vi "Create.vi"(8 "error in (no error)":errorcluster, 10 "gRPC ID in":T1) -> (0 "error out":errorcluster, 2 "gRPC ID out":T1, 3 "IMeasurementService out":refnum<class "IMeasurementService.lvclass">)   [LabVIEW 2020, in "MeasurementLink Measurement Server.lvlib" / "MeasurementServiceV2.lvclass"]
uses:
  MeasurementServiceV2.lvclass
  IMeasurementService/IMeasurementService.lvclass
  <vilib>/gRPC/LabVIEW gRPC Library/Shared/grpcId.ctl
  MeasurementLink Measurement Service Base V2/RPC Service/MeasurementService/MeasurementServiceBaseV2.lvclass
  \\tsclient\C/dev/measurementlink-labview/Source/Runtime/MeasurementLink Measurement Server/Classes/IMeasurementService/IMeasurementService.lvclass
  MeasurementServiceV2.lvclass/MeasurementServiceV2.ctl
  <vilib>/gRPC/LabVIEW gRPC Library/grpc-lvsupport-release.lvlib
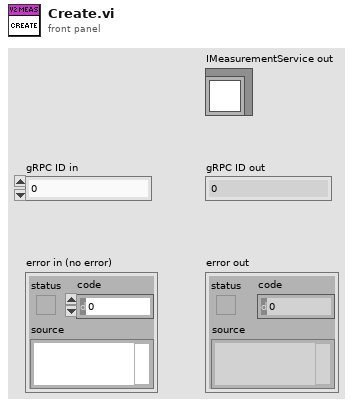
[diagram p1: front panel]
types:
  T1 = typedef "grpc-lvsupport-release.lvlib/grpcId.ctl" = u64
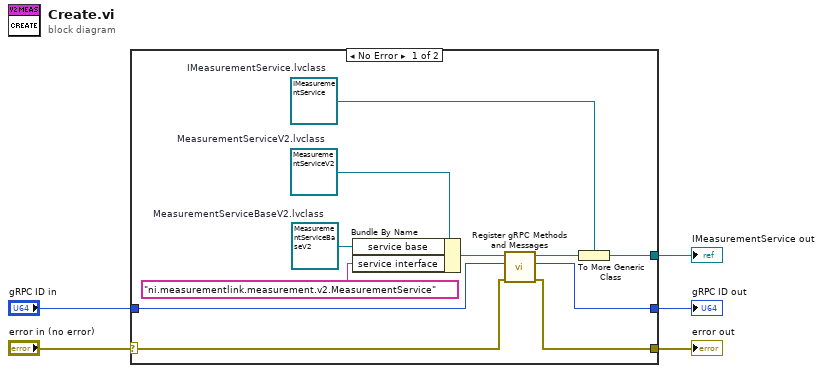
[diagram p0: block diagram]
diagram:
  n1 = case shown="No Error" "error in (no error)" {
    selector: "error in (no error)" -> [w8 w18]
    tunnel: [w7 w18] -> w4
    tunnel: [w14 _] -> w3
    tunnel: "gRPC ID in" -> [w9 w17]
    tunnel: [w6 w17] -> w1
    frame No Error {
      w12 = refnum<class "MeasurementServiceV2.lvclass"> refnum  # MeasurementServiceV2.lvclass
      w13 = refnum<class "IMeasurementService.lvclass"> refnum  # IMeasurementService.lvclass
      w16 = refnum<class "MeasurementServiceBaseV2.lvclass"> refnum  # MeasurementServiceBaseV2.lvclass
      n2 = Bundle By Name(cluster=w12, "service base"=w16, "service interface"="ni.measurementlink.measurement.v2.MeasurementService") -> (w11:refnum<class "MeasurementServiceV2.lvclass">)
      n3 = call "Register gRPC Methods and Messages.vi"("error in (no error)"=w8, "gRPC ID in"=w9, "MeasurementServiceV2 in"=w11) -> ("error out"=w7:errorcluster, "gRPC ID out"=w6:T1, "MeasurementServiceV2 out"=w10:refnum<class "MeasurementServiceV2.lvclass">)  [unwired: 6 in]
      n4 = To More Generic Class(target class=w13, reference=w10) -> (generic class reference=w14:refnum<class "IMeasurementService.lvclass">)
    }
    frame Error {
    }
  }
  "error out" <- w4
  "IMeasurementService out" <- w3
  "gRPC ID out" <- w1
